vi "microFPGA_camera_firepulse_time_addr_42_ctrl.vi"(0 "VISA resource name":refnum<visa-resource-name>, 2 "write or read":u16(ring) items=["read", "write"], 5 "camera_fire_pulse_time_WRITE":u32(slide) max=1048580 step=1 scale=0.0..1048575.0 scale format="%u us", 11 "error in (no error)":errorcluster) -> (4 "VISA resource name 2":refnum<visa-resource-name>, 6 "camera_fire_pulse_time_READ":u32(slide) max=65535 step=1 scale=0.0..1048575.0 scale format="%u us", 8 "value write confirm":bool, 10 "abort_wrong_input":bool, 15 "error out":errorcluster)   [LabVIEW 2018]
panel:
  out "mode read string answer":string
  out "mode read string":string
  out "mode write string":string
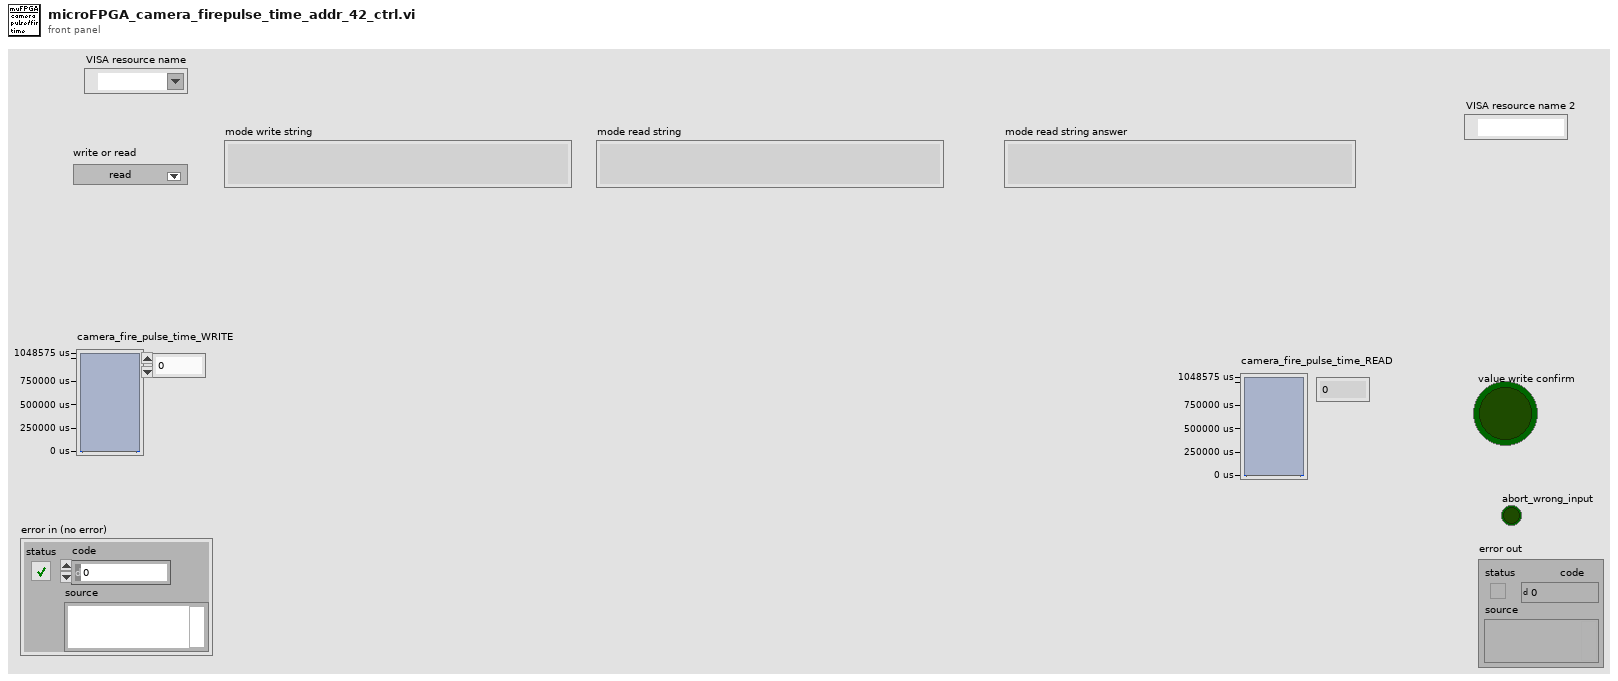
[diagram p1: front panel]
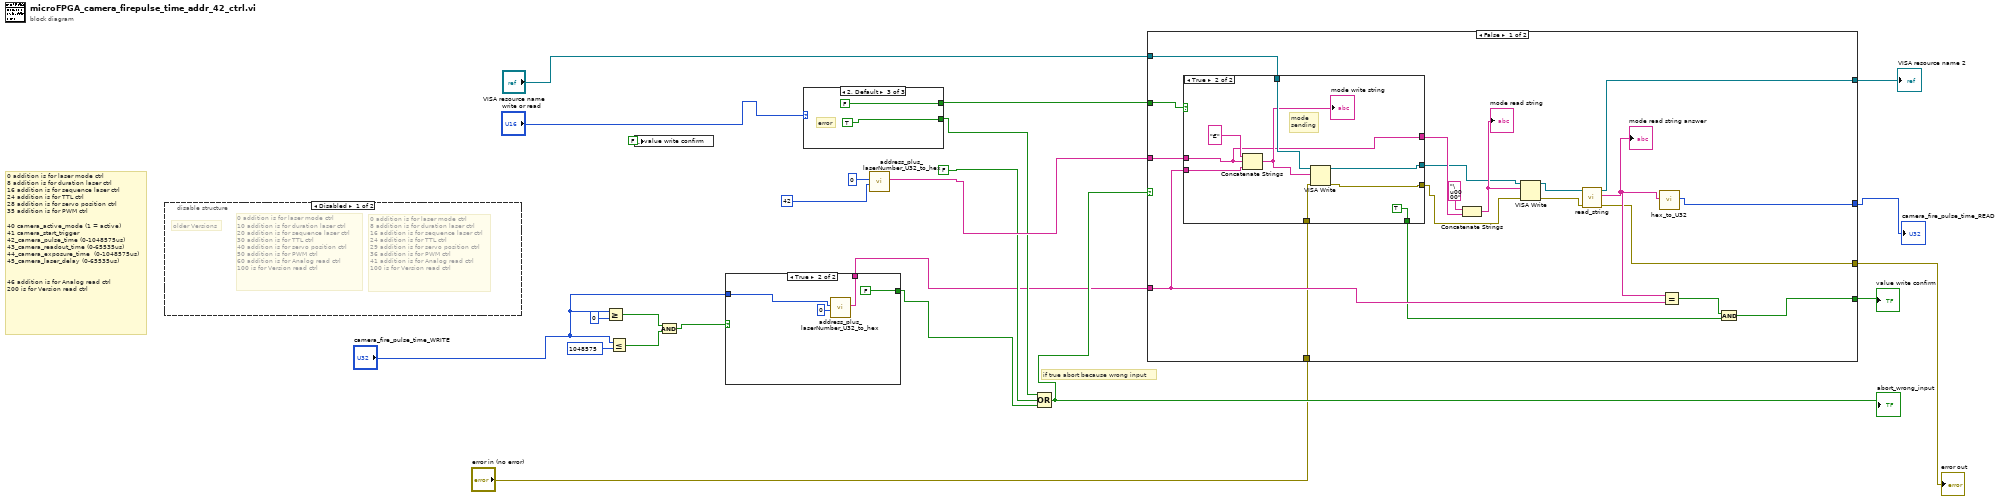
[diagram p0: block diagram]
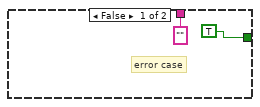
[diagram p3: hidden frame]
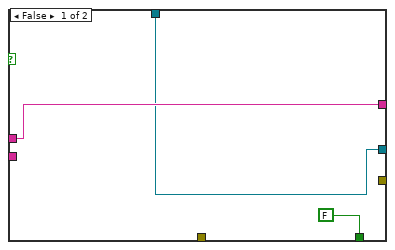
[diagram p4: hidden frame]
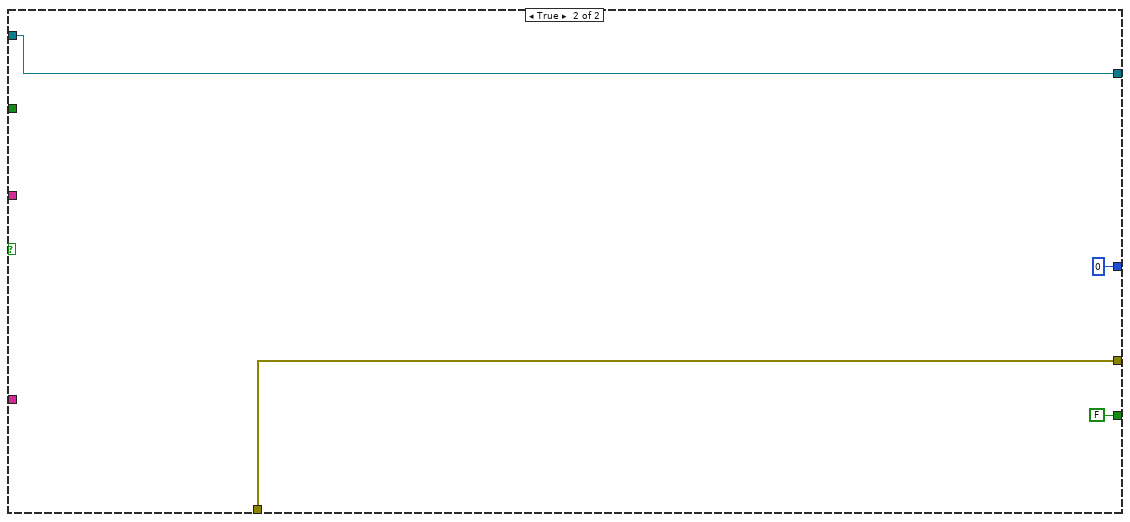
[diagram p5: hidden frame]
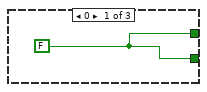
[diagram p6: hidden frame]
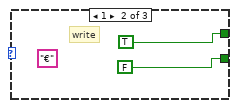
[diagram p7: hidden frame]
diagram:
  # "0 addition is for laser mode ctrl\n8 addition is for duration laser ctrl\n16 addition is for sequence laser ctrl\n24 addition is for TTL ctrl\n28 addition is for servo position ctrl\n35 addition is for PWM ctrl\n\n40 camera_active_mode (1 = active) \n41 camera_start_trigger\n42_camera_pulse_time (0-1048575us)\n43_camera_readout_time (0-65535us)\n44_camera_exposure_time  (0-1048575us)\n45_camera_laser_delay (0-65535us)\n\n\n46 addition is for Analog read ctrl\n200 is for Version read ctrl"
  # "if true abort because wrong input"
  n1 = disable-structure shown="Disabled" {
    frame Disabled {
      # "older Versions"
      # "0 addition is for laser mode ctrl\n8 addition is for duration laser ctrl\n16 addition is for sequence laser ctrl\n24 addition is for TTL ctrl\n29 addition is for servo position ctrl\n36 addition is for PWM ctrl\n41 addition is for Analog read ctrl\n100 is for Version read ctrl"
      # "0 addition is for laser mode ctrl\n10 addition is for duration laser ctrl\n20 addition is for sequence laser ctrl\n30 addition is for TTL ctrl\n40 addition is for servo position ctrl\n50 addition is for PWM ctrl\n60 addition is for Analog read ctrl\n100 is for Version read ctrl"
    }
    frame Enabled {
    }
  }
  n2 = Greater Or Equal?(x="camera_fire_pulse_time_WRITE", y=u32 0) -> (x >= y?=w8:bool)
  n3 = Less Or Equal?(x="camera_fire_pulse_time_WRITE", y=u32 1048575) -> (x <= y?=w7:bool)
  n4 = local write "value write confirm"(FALSE ("value confirm")) -> ()
  n5 = And(x=w8, y=w7) -> (x .and. y?=w6:bool)
  n6 = case shown="True" w6 {
    tunnel: "camera_fire_pulse_time_WRITE" -> [_ w28]
    tunnel: [TRUE FALSE] -> w5
    tunnel: ["" ("string 5") w26] -> w4
    frame False {
      # "error case"
    }
    frame True {
      n7 = call "address_plus_laserNumber_U32_to_hex.vi"("adress offset"=u32 0, "y 3"=w28) -> ("string 5"=w26:string)  [unwired: 8 in]
    }
  }
  n8 = case shown="2, Default" "write or read" {
    tunnel: [w30 TRUE FALSE] -> w20
    tunnel: [w30 FALSE TRUE] -> w18
    frame 0 {
      w30 = FALSE
    }
    frame 1 {
      (unwired) "€" ("hex")
      # "write"
    }
    frame 2, Default {
      # "error"
    }
  }
  n9 = call "address_plus_laserNumber_U32_to_hex.vi"("adress offset"=u32 42, "y 3"=u32 0) -> ("string 5"=w21:string)  [unwired: 8 in]
  n10 = Compound Arithmetic op=OR(w18, FALSE, w5) -> (w15:bool)
  "abort_wrong_input" <- w15
  n11 = case shown="False" w15 {
    tunnel: "VISA resource name" -> [w53 w67]
    tunnel: w21 -> [w50 _]
    tunnel: w20 -> [w44 _]
    tunnel: w4 -> [w42 _]
    tunnel: [w41 u32 0 ("U32")] -> w1
    tunnel: [w35 FALSE] -> w16
    tunnel: [w40 w67] -> w14
    tunnel: "error in (no error)" -> [w39 w66]
    tunnel: [w38 w66] -> w12
    frame False {
      n12 = case shown="True" w44 {
        tunnel: w50 -> [w56 w62]
        tunnel: w53 -> [w55 w64]
        tunnel: [w56 w62] -> w51
        tunnel: w42 -> [_ w61]
        tunnel: [w55 w60] -> w46
        tunnel: [_ w59] -> w45
        tunnel: w39 -> [_ w58]
        tunnel: [FALSE TRUE] -> w37
        frame False {
        }
        frame True {
          # "mode \nsending"
          n13 = Concatenate Strings("€" ("string"), w62, w61) -> (w63:string)
          "mode write string" <- w63
          n14 = VISA Write(VISA resource name=w64, write buffer=w63, error in (no error)=w58) -> (VISA resource name out=w60:refnum<visa-resource-name>, error out=w59:errorcluster)  [unwired: 1 out]
        }
      }
      n15 = Concatenate Strings("\u0000" ("string"), w51) -> (w49:string)
      "mode read string" <- w49
      n16 = VISA Write(VISA resource name=w46, write buffer=w49, error in (no error)=w45) -> (VISA resource name out=w48:refnum<visa-resource-name>, error out=w47:errorcluster)  [unwired: 1 out]
      n17 = call "read_string.vi"("error in (no error)"=w47, "VISA resource name 2"=w48) -> ("error out"=w38:errorcluster, "read buffer"=w43:string, "VISA resource name"=w40:refnum<visa-resource-name>)  [unwired: 7 in]
      "mode read string answer" <- w43
      n18 = call "hex_to_U32.vi"("hex"=w43) -> ("U32"=w41:u32)  [unwired: 9 in]
      n19 = Equal?(x=w43, y=w42) -> (x = y?=w36:bool)
      n20 = And(x=w36, y=w37) -> (x .and. y?=w35:bool)
    }
    frame True {
    }
  }
  "value write confirm" <- w16
  "VISA resource name 2" <- w14
  "error out" <- w12
  "camera_fire_pulse_time_READ" <- w1
